vi "tokenize_string.vi"(8 "error in (no error)":errorcluster, 10 "delimiter":string, 11 "input_string":string) -> (0 "error out":errorcluster, 3 "delimited_string []":string[](array[string]))   [LabVIEW 2015, in "lv-build.lvlib"]
uses:
  lv-build.lvlib
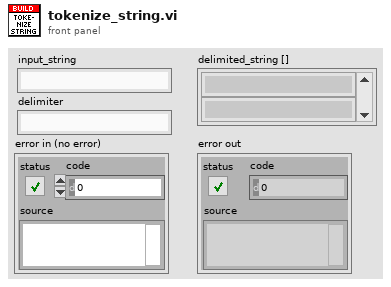
[diagram p1: front panel]
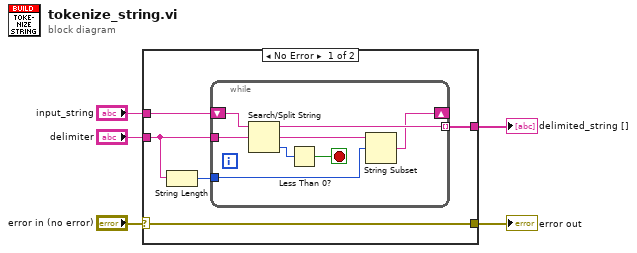
[diagram p0: block diagram]
diagram:
  n1 = case shown="No Error" "error in (no error)" {
    selector: "error in (no error)" -> [w7 w19]
    tunnel: "delimiter" -> [w10 _]
    tunnel: [w9 _] -> w4
    tunnel: "input_string" -> [w8 _]
    tunnel: [w7 w19] -> w1
    frame No Error {
      n2 = String Length(string=w10) -> (length=w6:i32)
      n3 = while {
        tunnel: [w18] -> w9 mode=indexing
        shift-right: [w14] -> _
        shift-left: w8 -> [w12]
        tunnel: w10 -> [w13]
        tunnel: w6 -> [w11]
        stop <- w17 stop-if-true
        n4 = Search/Split String(string=w12, search string/char (-)=w13) -> (substring before match=w18:string, match + rest of string=w15:string, offset of match=w16:i32)  [unwired: 1 in]
        n5 = Less Than 0?(x=w16) -> (x < 0?=w17:bool)
        n6 = String Subset(string=w15, offset (0)=w11) -> (substring=w14:string)  [unwired: 1 in]
      }
    }
    frame Error {
    }
  }
  "delimited_string []" <- w4
  "error out" <- w1
